vi "LabviewProgram.vi"() -> ()   [LabVIEW 2020]
uses:
  #typedefenum.ctl
  #typedefprogramdata.ctl
  #typedefcontrol.ctl
panel:
  in  "Czas na odpowiedŸ w sekundach":u16=5
  in  "Exit":bool caption="Learning"
  in  "Stop":bool caption="Learning"
  in  "Test":bool caption="Learning"
  in  "Learning":bool
  out "Angielski_Indicator":string caption="Angielski"
  out "Polski":string
  in  "Angielski_Write":string caption="Angielski"
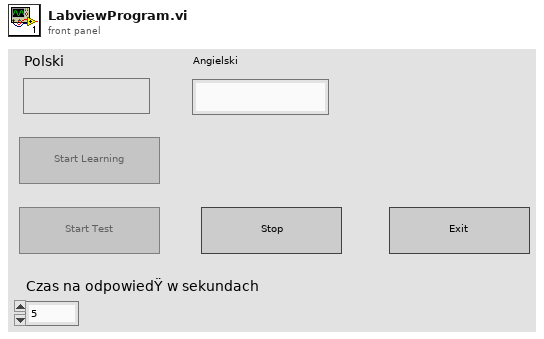
[diagram p1: front panel]
types:
  T1 = typedef "#typedefenum.ctl" = enum16{"Initialize", "Zero", "Learning_Polski", "Learning_Angielski", "Learning_Przerwa", "Test", "WynikTrue", "WynikFalse"}
  T2 = typedef "#typedefcontrol.ctl" = enum16{"Enabled", "Disabled", "Disabled and Grayed Out"}
  T3 = typedef "#typedefprogramdata.ctl" = cluster{"Slownik":string[][], "Iterator":i32}
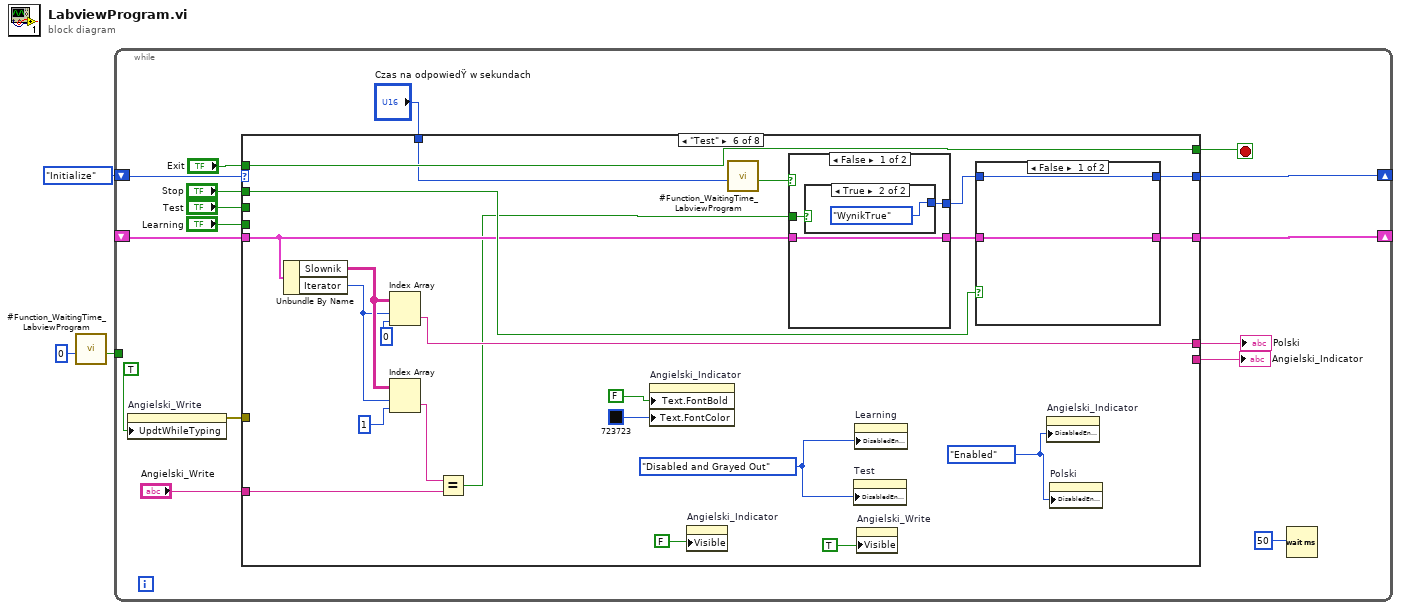
[diagram p0: block diagram]
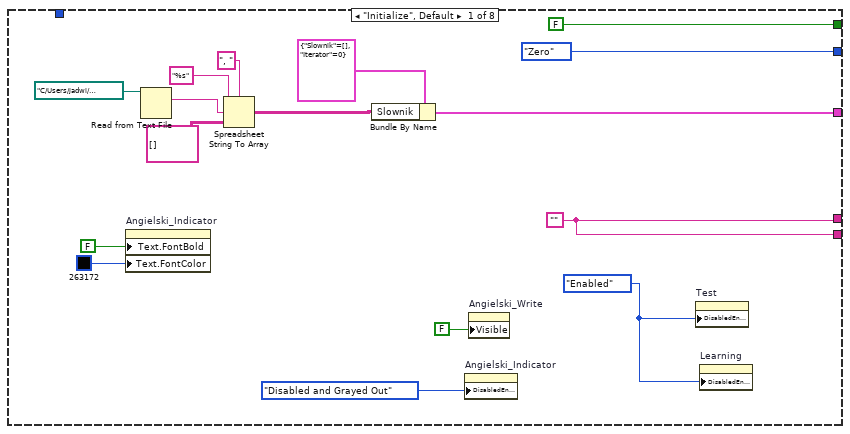
[diagram p2: hidden frame]
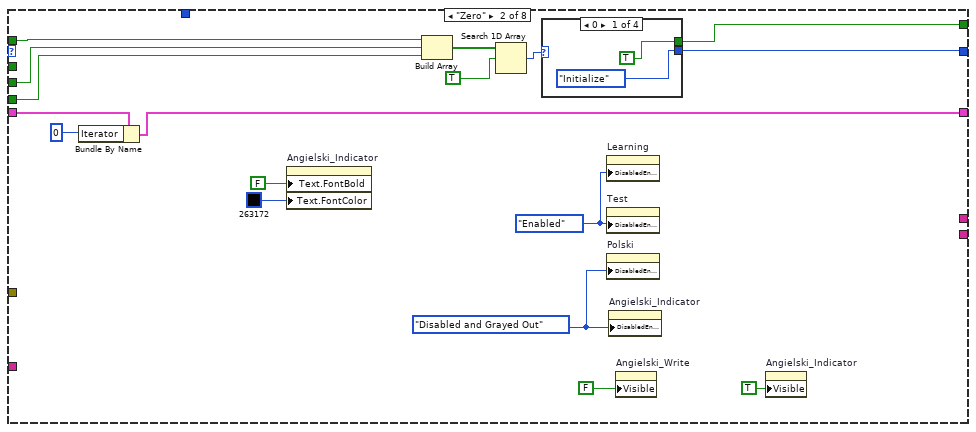
[diagram p3: hidden frame]
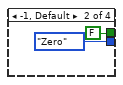
[diagram p4: hidden frame]
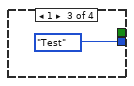
[diagram p5: hidden frame]
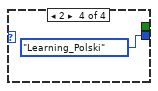
[diagram p6: hidden frame]
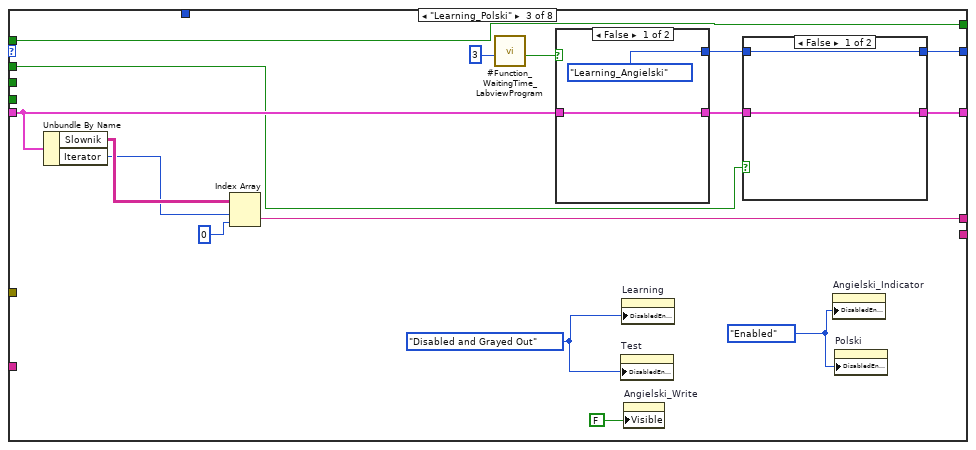
[diagram p7: hidden frame]
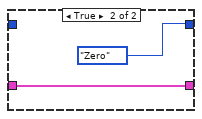
[diagram p8: hidden frame]
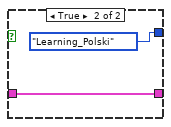
[diagram p9: hidden frame]
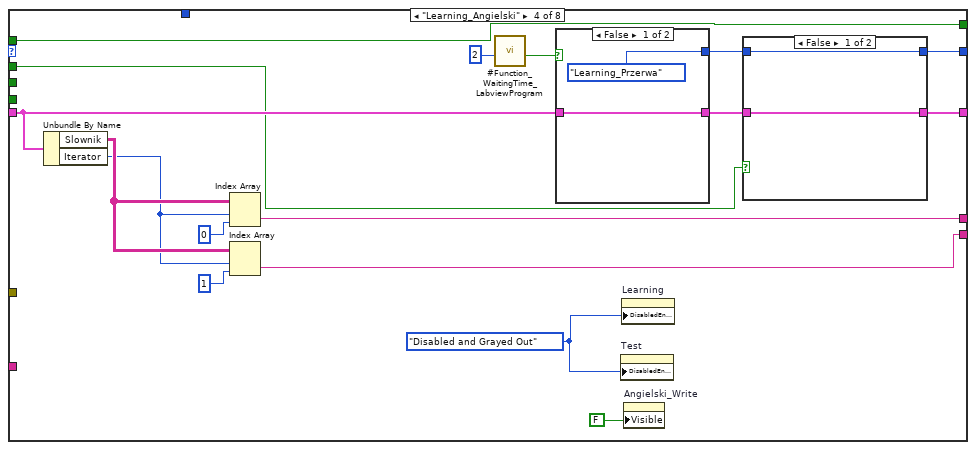
[diagram p10: hidden frame]
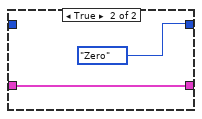
[diagram p11: hidden frame]
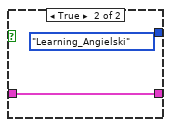
[diagram p12: hidden frame]
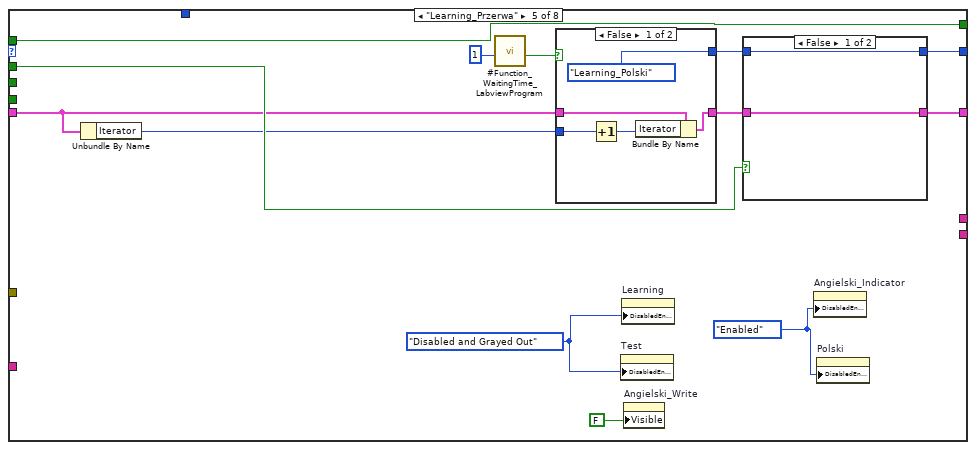
[diagram p13: hidden frame]
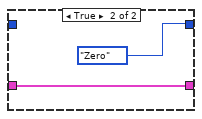
[diagram p14: hidden frame]
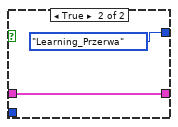
[diagram p15: hidden frame]
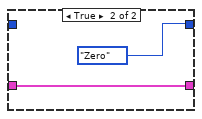
[diagram p16: hidden frame]
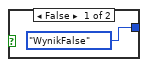
[diagram p17: hidden frame]
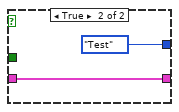
[diagram p18: hidden frame]
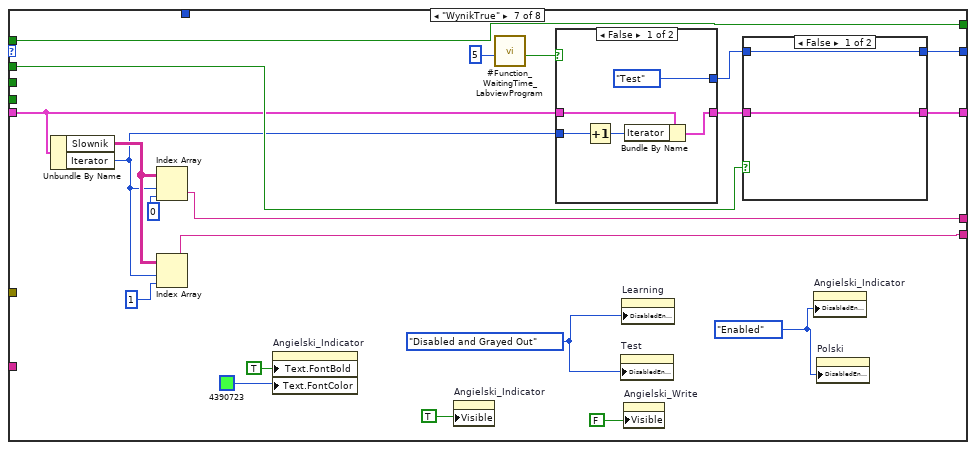
[diagram p19: hidden frame]
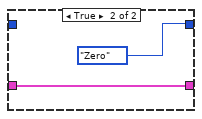
[diagram p20: hidden frame]
diagram:
  n1 = call "#Function_WaitingTime_LabviewProgram.vi"("Time"=0) -> ("Boolean"=w1:bool)  [unwired: 9 in, 1 out]
  n2 = while {
    shift-right: [w18] -> _
    shift-left: _ -> [w15]
    shift-right: [w16] -> _
    shift-left: #typedefenum."Initialize" -> [w17]
    tunnel: w1 -> [_]
    stop <- w19 stop-if-true
    n3 = property on="Angielski_Write" class="Str"("UpdtWhileTyping"=TRUE ("Update While Typing?")) -> (error out=w5:errorcluster)  [unwired: 2 in, 1 out]
    n4 = case shown="\"Test\"" w17 {
      tunnel: [FALSE w43 w65 w92 w116 w151 w182 w213] -> w19
      tunnel: [w28 w40 w63 w90 w115 w150 w181 w212] -> w18
      tunnel: [#typedefenum."Zero" w52 w61 w88 w113 w148 w179 w210] -> w16
      tunnel: w15 -> [_ w42 w70 w95 w110 w143 w174 w205]
      tunnel: "Exit" -> [_ w49 w65 w92 w116 w151 w182 w213]
      tunnel: "Test" -> [_ w48 _ _ _ _ _ _]
      tunnel: "Learning" -> [_ w47 _ _ _ _ _ _]
      tunnel: [w23 _ w66 w93 _ w141 w172 w203] -> w10
      tunnel: [w23 _ _ w85 _ _ w169 w199] -> w9
      tunnel: "Stop" -> [_ _ w64 w91 w111 w146 w177 w208]
      tunnel: "Angielski_Write" -> [_ _ _ _ _ w133 _ w199]
      tunnel: w5 -> [_ _ _ _ _ _ _ _]
      tunnel: "Czas na odpowiedŸ w sekundach" -> [_ _ _ _ _ w132 _ _]
      frame "Initialize", Default {
        w22 = #typedefcontrol."Enabled"
        w23 = ""
        n5 = property on="Angielski_Indicator" class="Str"("Text.FontBold"=FALSE, "Text.FontColor"=u32 263172) -> ()  [unwired: 2 in, 2 out]
        n6 = Read from Text File(file (use dialog)=path "C:/Users/jadwi/Documents/Slownik.txt") -> (text=w33:string)  [unwired: 3 in, 3 out]
        n7 = Spreadsheet String To Array(delimiter (Tab)=", ", format string="%s", spreadsheet string=w33, array type (2D Dbl)=string[][] []) -> (array=w24:string[][])
        n8 = Bundle By Name(cluster=T3 {"Slownik"=[], "Iterator"=0}, "Slownik"=w24) -> (w28:T3)
        n9 = property on="Angielski_Indicator" class="Str"("DisabledEnum"=#typedefcontrol."Disabled and Grayed Out") -> ()  [unwired: 2 in, 2 out]
        n10 = property on="Angielski_Write" class="Str"("Visible"=FALSE) -> ()  [unwired: 2 in, 2 out]
        n11 = property on="Test" class="Bool"("DisabledEnum"=w22) -> ()  [unwired: 2 in, 2 out]
        n12 = property on="Learning" class="Bool"("DisabledEnum"=w22) -> ()  [unwired: 2 in, 2 out]
      }
      frame "Zero" {
        w39 = #typedefcontrol."Enabled"
        w50 = #typedefcontrol."Disabled and Grayed Out"
        n13 = Bundle By Name(cluster=w42, "Iterator"=0) -> (w40:T3)
        n14 = property on="Angielski_Indicator" class="Str"("Text.FontBold"=FALSE, "Text.FontColor"=u32 263172) -> ()  [unwired: 2 in, 2 out]
        n15 = Build Array(w49, w48, w47) -> (w46:bool[])
        n16 = Search 1D Array(1D array=w46, element=TRUE) -> (index of element=w44:i32)  [unwired: 1 in]
        n17 = case shown="0" w44 {
          tunnel: [#typedefenum."Initialize" #typedefenum."Zero" #typedefenum."Test" #typedefenum."Learning_Polski"] -> w52
          tunnel: [TRUE FALSE _ _] -> w43
          frame 0 {
          }
          frame -1, Default {
          }
          frame 1 {
          }
          frame 2 {
          }
        }
        n18 = property on="Learning" class="Bool"("DisabledEnum"=w39) -> ()  [unwired: 2 in, 2 out]
        n19 = property on="Test" class="Bool"("DisabledEnum"=w39) -> ()  [unwired: 2 in, 2 out]
        n20 = property on="Polski" class="Str"("DisabledEnum"=w50) -> ()  [unwired: 2 in, 2 out]
        n21 = property on="Angielski_Indicator" class="Str"("DisabledEnum"=w50) -> ()  [unwired: 2 in, 2 out]
        n22 = property on="Angielski_Write" class="Str"("Visible"=FALSE) -> ()  [unwired: 2 in, 2 out]
        n23 = property on="Angielski_Indicator" class="Str"("Visible"=TRUE) -> ()  [unwired: 2 in, 2 out]
      }
      frame "Learning_Polski" {
        w59 = #typedefcontrol."Enabled"
        w74 = #typedefcontrol."Disabled and Grayed Out"
        n24 = Unbundle By Name(w70) -> ("Slownik"=w69:string[][], "Iterator"=w68:i32)
        n25 = Index Array(array=w69, index (row)=w68, index (col)=0) -> (element=w66:string)
        n26 = call "#Function_WaitingTime_LabviewProgram.vi"("Time"=3) -> ("Boolean"=w71:bool)  [unwired: 9 in, 1 out]
        n27 = case shown="False" w71 {
          tunnel: [#typedefenum."Learning_Angielski" #typedefenum."Learning_Polski"] -> w60
          tunnel: [w79 w81] -> w62
          tunnel: w70 -> [w79 w81]
          frame False {
          }
          frame True {
          }
        }
        n28 = property on="Test" class="Bool"("DisabledEnum"=w74) -> ()  [unwired: 2 in, 2 out]
        n29 = property on="Learning" class="Bool"("DisabledEnum"=w74) -> ()  [unwired: 2 in, 2 out]
        n30 = property on="Angielski_Write" class="Str"("Visible"=FALSE) -> ()  [unwired: 2 in, 2 out]
        n31 = case shown="False" w64 {
          tunnel: [w76 w78] -> w63
          tunnel: w62 -> [w76 w78]
          tunnel: [w75 #typedefenum."Zero"] -> w61
          tunnel: w60 -> [w75 _]
          frame False {
          }
          frame True {
          }
        }
        n32 = property on="Angielski_Indicator" class="Str"("DisabledEnum"=w59) -> ()  [unwired: 2 in, 2 out]
        n33 = property on="Polski" class="Str"("DisabledEnum"=w59) -> ()  [unwired: 2 in, 2 out]
      }
      frame "Learning_Angielski" {
        w99 = #typedefcontrol."Disabled and Grayed Out"
        n34 = Unbundle By Name(w95) -> ("Slownik"=w84:string[][], "Iterator"=w83:i32)
        n35 = Index Array(array=w84, index (row)=w83, index (col)=0) -> (element=w93:string)
        n36 = Index Array(array=w84, index (row)=w83, index (col)=1) -> (element=w85:string)
        n37 = call "#Function_WaitingTime_LabviewProgram.vi"("Time"=2) -> ("Boolean"=w96:bool)  [unwired: 9 in, 1 out]
        n38 = case shown="False" w96 {
          tunnel: [#typedefenum."Learning_Przerwa" #typedefenum."Learning_Angielski"] -> w87
          tunnel: [w104 w106] -> w89
          tunnel: w95 -> [w104 w106]
          frame False {
          }
          frame True {
          }
        }
        n39 = property on="Test" class="Bool"("DisabledEnum"=w99) -> ()  [unwired: 2 in, 2 out]
        n40 = property on="Learning" class="Bool"("DisabledEnum"=w99) -> ()  [unwired: 2 in, 2 out]
        n41 = property on="Angielski_Write" class="Str"("Visible"=FALSE) -> ()  [unwired: 2 in, 2 out]
        n42 = case shown="False" w91 {
          tunnel: [w101 w103] -> w90
          tunnel: w89 -> [w101 w103]
          tunnel: [w100 #typedefenum."Zero"] -> w88
          tunnel: w87 -> [w100 _]
          frame False {
          }
          frame True {
          }
        }
      }
      frame "Learning_Przerwa" {
        w108 = #typedefcontrol."Enabled"
        w120 = #typedefcontrol."Disabled and Grayed Out"
        n43 = Unbundle By Name(w110) -> ("Iterator"=w109:i32)
        n44 = call "#Function_WaitingTime_LabviewProgram.vi"("Time"=1) -> ("Boolean"=w117:bool)  [unwired: 9 in, 1 out]
        n45 = case shown="False" w117 {
          tunnel: [#typedefenum."Learning_Polski" #typedefenum."Learning_Przerwa"] -> w112
          tunnel: [w126 w130] -> w114
          tunnel: w110 -> [w127 w130]
          tunnel: w109 -> [w125 _]
          frame False {
            n46 = Increment(x=w125) -> (x+1=w128:i32)
            n47 = Bundle By Name(cluster=w127, "Iterator"=w128) -> (w126:T3)
          }
          frame True {
          }
        }
        n48 = property on="Test" class="Bool"("DisabledEnum"=w120) -> ()  [unwired: 2 in, 2 out]
        n49 = property on="Learning" class="Bool"("DisabledEnum"=w120) -> ()  [unwired: 2 in, 2 out]
        n50 = property on="Angielski_Write" class="Str"("Visible"=FALSE) -> ()  [unwired: 2 in, 2 out]
        n51 = case shown="False" w111 {
          tunnel: [w122 w124] -> w115
          tunnel: w114 -> [w122 w124]
          tunnel: [w121 #typedefenum."Zero"] -> w113
          tunnel: w112 -> [w121 _]
          frame False {
          }
          frame True {
          }
        }
        n52 = property on="Angielski_Indicator" class="Str"("DisabledEnum"=w108) -> ()  [unwired: 2 in, 2 out]
        n53 = property on="Polski" class="Str"("DisabledEnum"=w108) -> ()  [unwired: 2 in, 2 out]
      }
      frame "Test" {
        w145 = #typedefcontrol."Enabled"
        w154 = #typedefcontrol."Disabled and Grayed Out"
        n54 = Unbundle By Name(w143) -> ("Slownik"=w140:string[][], "Iterator"=w138:i32)
        n55 = Index Array(array=w140, index (row)=w138, index (col)=0) -> (element=w141:string)
        n56 = Index Array(array=w140, index (row)=w138, index (col)=1) -> (element=w137:string)
        n57 = Equal?(x=w137, y=w133) -> (x = y?=w136:bool)
        n58 = property on="Angielski_Indicator" class="Str"("Text.FontBold"=FALSE, "Text.FontColor"=u32 723723) -> ()  [unwired: 2 in, 2 out]
        n59 = property on="Angielski_Indicator" class="Str"("Visible"=FALSE) -> ()  [unwired: 2 in, 2 out]
        n60 = call "#Function_WaitingTime_LabviewProgram.vi"("Time"=w132) -> ("Boolean"=w152:bool)  [unwired: 9 in, 1 out]
        n61 = case shown="False" w152 {
          tunnel: [w159 #typedefenum."Test"] -> w147
          tunnel: [w161 w164] -> w149
          tunnel: w143 -> [w161 w164]
          tunnel: w136 -> [w160 _]
          frame False {
            n62 = case shown="True" w160 {
              tunnel: [#typedefenum."WynikFalse" #typedefenum."WynikTrue"] -> w159
              frame False {
              }
              frame True {
              }
            }
          }
          frame True {
          }
        }
        n63 = property on="Test" class="Bool"("DisabledEnum"=w154) -> ()  [unwired: 2 in, 2 out]
        n64 = property on="Learning" class="Bool"("DisabledEnum"=w154) -> ()  [unwired: 2 in, 2 out]
        n65 = property on="Angielski_Write" class="Str"("Visible"=TRUE) -> ()  [unwired: 2 in, 2 out]
        n66 = case shown="False" w146 {
          tunnel: [w156 w158] -> w150
          tunnel: w149 -> [w156 w158]
          tunnel: [w155 #typedefenum."Zero"] -> w148
          tunnel: w147 -> [w155 _]
          frame False {
          }
          frame True {
          }
        }
        n67 = property on="Angielski_Indicator" class="Str"("DisabledEnum"=w145) -> ()  [unwired: 2 in, 2 out]
        n68 = property on="Polski" class="Str"("DisabledEnum"=w145) -> ()  [unwired: 2 in, 2 out]
      }
      frame "WynikTrue" {
        w176 = #typedefcontrol."Enabled"
        w186 = #typedefcontrol."Disabled and Grayed Out"
        n69 = Unbundle By Name(w174) -> ("Slownik"=w171:string[][], "Iterator"=w167:i32)
        n70 = Index Array(array=w171, index (row)=w167, index (col)=0) -> (element=w172:string)
        n71 = Index Array(array=w171, index (row)=w167, index (col)=1) -> (element=w169:string)
        n72 = property on="Angielski_Indicator" class="Str"("Text.FontBold"=TRUE, "Text.FontColor"=u32 4390723) -> ()  [unwired: 2 in, 2 out]
        n73 = property on="Angielski_Indicator" class="Str"("Visible"=TRUE) -> ()  [unwired: 2 in, 2 out]
        n74 = call "#Function_WaitingTime_LabviewProgram.vi"("Time"=5) -> ("Boolean"=w183:bool)  [unwired: 9 in, 1 out]
        n75 = case shown="False" w183 {
          tunnel: [#typedefenum."Test" #typedefenum."WynikTrue"] -> w178
          tunnel: [w193 w196] -> w180
          tunnel: w174 -> [w194 w196]
          tunnel: w167 -> [w191 _]
          frame False {
            n76 = Increment(x=w191) -> (x+1=w192:i32)
            n77 = Bundle By Name(cluster=w194, "Iterator"=w192) -> (w193:T3)
          }
          frame True {
          }
        }
        n78 = property on="Test" class="Bool"("DisabledEnum"=w186) -> ()  [unwired: 2 in, 2 out]
        n79 = property on="Learning" class="Bool"("DisabledEnum"=w186) -> ()  [unwired: 2 in, 2 out]
        n80 = property on="Angielski_Write" class="Str"("Visible"=FALSE) -> ()  [unwired: 2 in, 2 out]
        n81 = case shown="False" w177 {
          tunnel: [w188 w190] -> w181
          tunnel: w180 -> [w188 w190]
          tunnel: [w187 #typedefenum."Zero"] -> w179
          tunnel: w178 -> [w187 _]
          frame False {
          }
          frame True {
          }
        }
        n82 = property on="Angielski_Indicator" class="Str"("DisabledEnum"=w176) -> ()  [unwired: 2 in, 2 out]
        n83 = property on="Polski" class="Str"("DisabledEnum"=w176) -> ()  [unwired: 2 in, 2 out]
      }
      frame "WynikFalse" {
        w207 = #typedefcontrol."Enabled"
        w217 = #typedefcontrol."Disabled and Grayed Out"
        n84 = Unbundle By Name(w205) -> ("Slownik"=w202:string[][], "Iterator"=w200:i32)
        n85 = Index Array(array=w202, index (row)=w200, index (col)=0) -> (element=w203:string)
        n86 = property on="Angielski_Indicator" class="Str"("Text.FontBold"=TRUE, "Text.FontColor"=u32 16711680) -> ()  [unwired: 2 in, 2 out]
        n87 = property on="Angielski_Indicator" class="Str"("Visible"=TRUE) -> ()  [unwired: 2 in, 2 out]
        n88 = call "#Function_WaitingTime_LabviewProgram.vi"("Time"=5) -> ("Boolean"=w214:bool)  [unwired: 9 in, 1 out]
        n89 = case shown="False" w214 {
          tunnel: [#typedefenum."Test" #typedefenum."WynikFalse"] -> w209
          tunnel: [w224 w227] -> w211
          tunnel: w205 -> [w225 w227]
          tunnel: w200 -> [w222 _]
          frame False {
            n90 = Increment(x=w222) -> (x+1=w223:i32)
            n91 = Bundle By Name(cluster=w225, "Iterator"=w223) -> (w224:T3)
          }
          frame True {
          }
        }
        n92 = property on="Test" class="Bool"("DisabledEnum"=w217) -> ()  [unwired: 2 in, 2 out]
        n93 = property on="Learning" class="Bool"("DisabledEnum"=w217) -> ()  [unwired: 2 in, 2 out]
        n94 = property on="Angielski_Write" class="Str"("Visible"=FALSE) -> ()  [unwired: 2 in, 2 out]
        n95 = case shown="False" w208 {
          tunnel: [w219 w221] -> w212
          tunnel: w211 -> [w219 w221]
          tunnel: [w218 #typedefenum."Zero"] -> w210
          tunnel: w209 -> [w218 _]
          frame False {
          }
          frame True {
          }
        }
        n96 = property on="Angielski_Indicator" class="Str"("DisabledEnum"=w207) -> ()  [unwired: 2 in, 2 out]
        n97 = property on="Polski" class="Str"("DisabledEnum"=w207) -> ()  [unwired: 2 in, 2 out]
      }
    }
    "Polski" <- w10
    "Angielski_Indicator" <- w9
    n98 = Wait (ms)(milliseconds to wait=u32 50) -> ()  [unwired: 1 out]
  }
